vi "Msg EnQ.vi"(9 "Msg":refnum<class "Msg.lvclass">, 10 "Msg Q":refnum<class "Msg Q.lvclass">, 11 "Normal Msg EnQ in":refnum<class "Normal Msg EnQ.lvclass">) -> (0 "error out":errorcluster)   [LabVIEW 2021, in "AAM.lvlib" / "Normal Msg EnQ.lvclass"]
uses:
  Normal Msg EnQ.lvclass
  Msg/Msg.lvclass
  Msg Q/Msg Q.lvclass
  Msg Q/Msg Q.lvclass/Msg Q.ctl
  Msg Q/Read Msg Q.vi
  Normal Msg EnQ.lvclass/Normal Msg EnQ.ctl
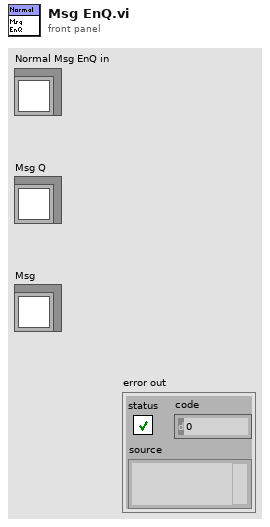
[diagram p1: front panel]
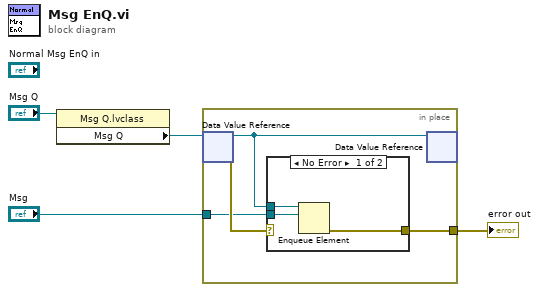
[diagram p0: block diagram]
diagram:
  n1 = property class="Msg Q.lvclass"(reference="Msg Q") -> ("Msg Q"=w4:refnum<data-value>)  [unwired: 1 in, 2 out]
  n2 = in-place {
    in-place-border: [w7] -> w3
    in-place-border: "Msg" -> [w6]
    n3 = in-place-dvr #1(w4) -> (w5:refnum<queue>, w8:errorcluster)
    n4 = case shown="No Error" w8 {
      selector: w8 -> [_ w12]
      tunnel: [w11 w12] -> w7
      tunnel: w6 -> [w9 _]
      tunnel: w5 -> [w10 _]
      frame No Error {
        n5 = Enqueue Element(queue=w10, element=w9) -> (error out=w11:errorcluster)  [unwired: 2 in, 2 out]
      }
      frame Error {
      }
    }
    n6 = in-place-dvr #1(w5) -> ()  [unwired: 2 out]
  }
  "error out" <- w3
